vi "Hit Detect.vi"(7 "Visible only? [T]":bool=TRUE, 8 "error in (no error)":errorcluster, 10 "Coords":T1, 11 "Interaction By Refererence in":refnum<class "Interaction By Refererence.lvclass">) -> (0 "error out":errorcluster, 1 "Hit?":bool, 2 "In Object":string[](array[string]), 3 "Interaction By Refererence out":refnum<class "Interaction By Refererence.lvclass">)   [LabVIEW 2021, in "Interaction By Refererence.lvclass"]
uses:
  Interaction By Refererence.lvclass
  <vilib>/Utility/miscctls.llb/LVPoint32TypeDef.ctl
  Interaction By Refererence.lvclass/Interaction By Refererence.ctl
  IContainer/Interaction/Interaction.lvclass
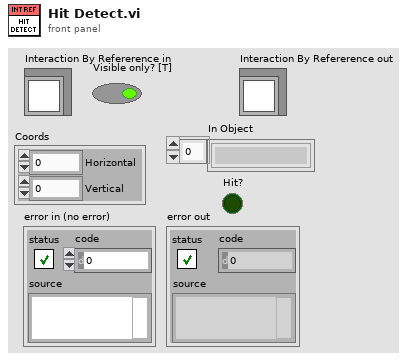
[diagram p1: front panel]
types:
  T1 = typedef "LVPoint32TypeDef.ctl" = cluster{"Horizontal":i32, "Vertical":i32}
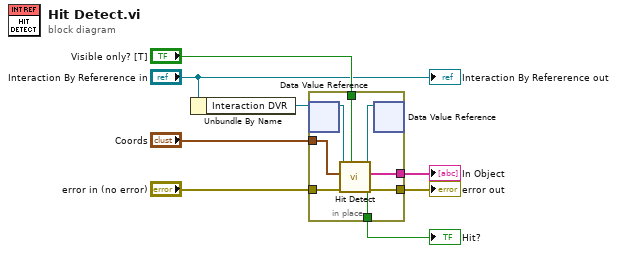
[diagram p0: block diagram]
diagram:
  n1 = Unbundle By Name("Interaction By Refererence in") -> ("Interaction DVR"=w3:refnum<data-value>)
  n2 = in-place {
    in-place-border: [w15] -> w7
    in-place-border: [w14] -> w2
    in-place-border: "error in (no error)" -> [w16]
    in-place-border: "Coords" -> [w10]
    in-place-border: "Visible only? [T]" -> [w11]
    in-place-border: [w9] -> w1
    n3 = in-place-dvr #1(w3) -> (w13:refnum<class "Interaction.lvclass">)  [unwired: 1 out]
    n4 = call-dynamic "Hit Detect.vi"("Visible only? [T]"=w11, "error in (no error)"=w16, "Coords"=w10, "IContainer in"=w13) -> ("error out"=w15:errorcluster, "Hit?"=w9:bool, "In Object"=w14:string[], "IContainer out"=w12:refnum<class "Interaction.lvclass">)  [unwired: 4 in]
    n5 = in-place-dvr #1(w12) -> ()  [unwired: 2 out]
  }
  "error out" <- w7
  "In Object" <- w2
  "Hit?" <- w1
  "Interaction By Refererence out" <- "Interaction By Refererence in"
